vi "CreateTriggerOutputNode.vi"(7 "DOM Document":refnum<k20>, 8 "Error In":errorcluster, 11 "Trigger Output Configuration":T1={"Type"=enum."None", "Delay (ms)"=0, "Digital IO Line (1-14)"=1, "Digital IO Mode"=enum."Falling", "Digital IO Pulse Width (sec)"=0.0001} {"Digital IO Line (1-14)" min=1 max=14 step=1}) -> (0 "Error Out":errorcluster, 3 "Trigger Output Node":refnum<k20>)   [LabVIEW 2012]
uses:
  TriggerOutputConfiguration.ctl
  TriggerOutputType.ctl
  driver/Public/Controls/TriggerMode.ctl
  libs/LV-Utilities/LV-Utilities.lvlib
  driver/Keithley-2602.lvlib
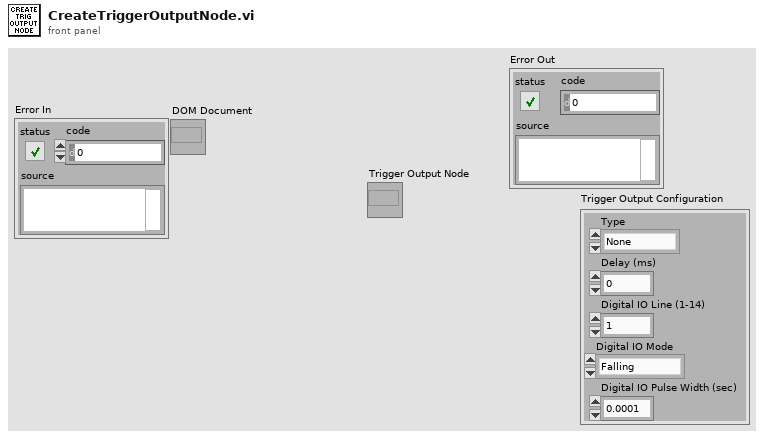
[diagram p1: front panel]
types:
  T1 = typedef "TriggerOutputConfiguration.ctl" = cluster{"Type":T2, "Delay (ms)":u32, "Digital IO Line (1-14)":u8, "Digital IO Mode":T3, "Digital IO Pulse Width (sec)":dbl}
  T2 = typedef "TriggerOutputType.ctl" = enum16{"None", "Digital IO", "Bus"}
  T3 = typedef "Keithley-2602.lvlib/TriggerMode.ctl" = enum16{"Falling", "Rising", "Either", "Synchronous"}
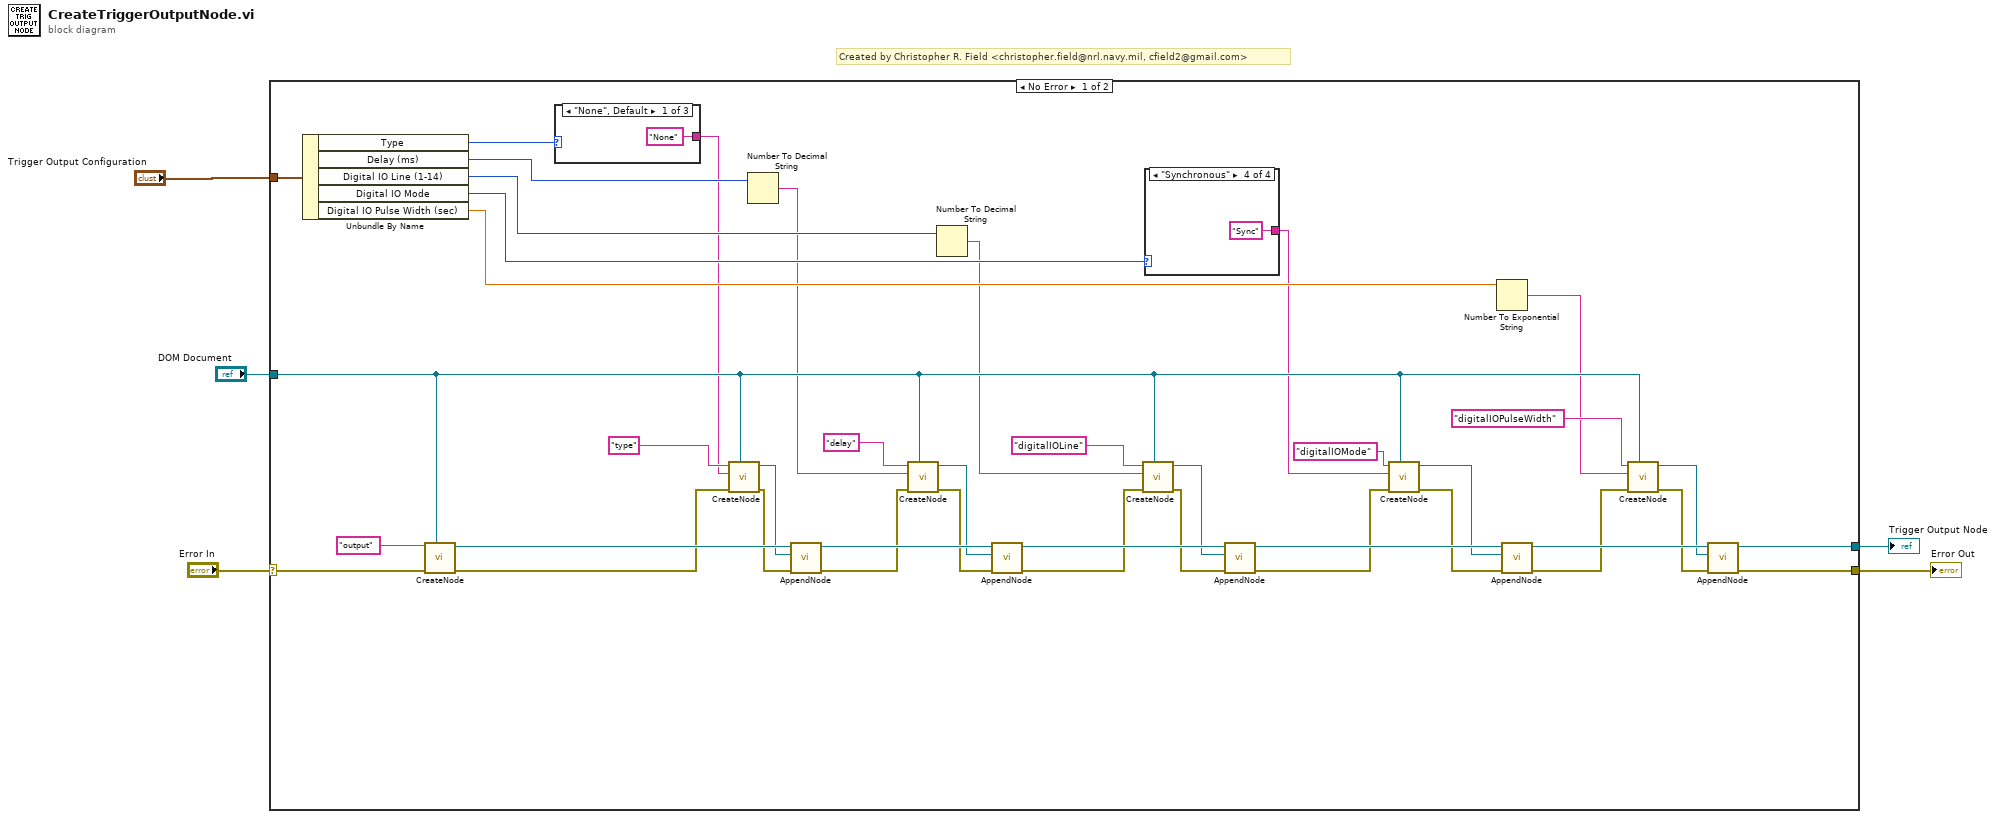
[diagram p0: block diagram]
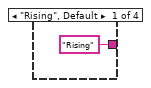
[diagram p2: hidden frame]
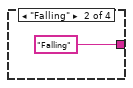
[diagram p3: hidden frame]
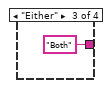
[diagram p4: hidden frame]
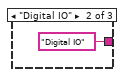
[diagram p5: hidden frame]
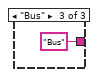
[diagram p6: hidden frame]
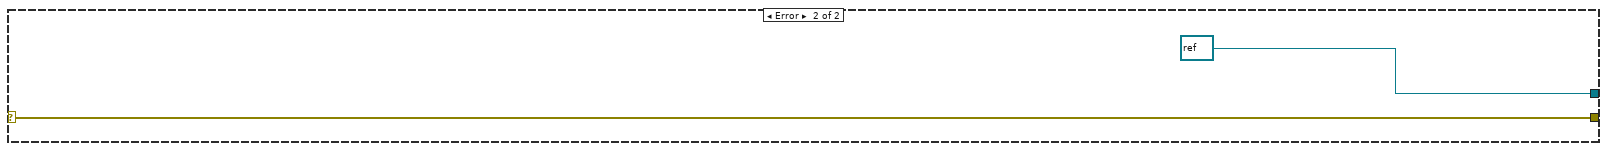
[diagram p7: hidden frame]
diagram:
  # "Created by Christopher R. Field <christopher.field@nrl.navy.mil, cfield2@gmail.com>"
  n1 = case shown="No Error" "Error In" {
    selector: "Error In" -> [w40 w55]
    tunnel: "DOM Document" -> [w26 _]
    tunnel: [w33 refnum<k20> refnum ("Wirings Node 2")] -> w3
    tunnel: [w32 w55] -> w2
    tunnel: "Trigger Output Configuration" -> [w45 _]
    frame No Error {
      n2 = Unbundle By Name(w45) -> ("Type"=w46:T2, "Delay (ms)"=w41:u32, "Digital IO Line (1-14)"=w44:u8, "Digital IO Mode"=w43:T3, "Digital IO Pulse Width (sec)"=w42:dbl)
      n3 = call "CreateNode.vi"("DOM Document"=w26, "Error In"=w40, "Tag Name"="output") -> ("Error out"=w25:errorcluster, "Node"=w38:refnum<k20>)  [unwired: 7 in]
      n4 = case shown="\"None\", Default" w46 {
        tunnel: ["None" "Digital IO" "Bus"] -> w10
        frame "None", Default {
        }
        frame "Digital IO" {
        }
        frame "Bus" {
        }
      }
      n5 = call "CreateNode.vi"("DOM Document"=w26, "Error In"=w25, "Text"=w10, "Tag Name"="type") -> ("Error out"=w24:errorcluster, "Node"=w11:refnum<k20>)  [unwired: 6 in]
      n6 = Number To Decimal String(number=w41) -> (decimal integer string=w9:string)  [unwired: 1 in]
      n7 = call "AppendNode.vi"("Error In"=w24, "Child Node"=w11, "Parent Node In"=w38) -> ("Error Out"=w23:errorcluster, "Parent Node Out"=w37:refnum<k20>)  [unwired: 7 in]
      n8 = call "CreateNode.vi"("DOM Document"=w26, "Error In"=w23, "Text"=w9, "Tag Name"="delay") -> ("Error out"=w22:errorcluster, "Node"=w12:refnum<k20>)  [unwired: 6 in]
      n9 = Number To Decimal String(number=w44) -> (decimal integer string=w8:string)  [unwired: 1 in]
      n10 = call "AppendNode.vi"("Error In"=w22, "Child Node"=w12, "Parent Node In"=w37) -> ("Error Out"=w21:errorcluster, "Parent Node Out"=w36:refnum<k20>)  [unwired: 7 in]
      n11 = call "CreateNode.vi"("DOM Document"=w26, "Error In"=w21, "Text"=w8, "Tag Name"="digitalIOLine" ("Text")) -> ("Error out"=w20:errorcluster, "Node"=w13:refnum<k20>)  [unwired: 6 in]
      n12 = case shown="\"Synchronous\"" w43 {
        tunnel: ["Rising" "Falling" "Both" "Sync"] -> w7
        frame "Rising", Default {
        }
        frame "Falling" {
        }
        frame "Either" {
        }
        frame "Synchronous" {
        }
      }
      n13 = call "AppendNode.vi"("Error In"=w20, "Child Node"=w13, "Parent Node In"=w36) -> ("Error Out"=w19:errorcluster, "Parent Node Out"=w35:refnum<k20>)  [unwired: 7 in]
      n14 = call "CreateNode.vi"("DOM Document"=w26, "Error In"=w19, "Text"=w7, "Tag Name"="digitalIOMode") -> ("Error out"=w18:errorcluster, "Node"=w14:refnum<k20>)  [unwired: 6 in]
      n15 = Number To Exponential String(number=w42) -> (E-format string=w6:string)  [unwired: 3 in]
      n16 = call "AppendNode.vi"("Error In"=w18, "Child Node"=w14, "Parent Node In"=w35) -> ("Error Out"=w17:errorcluster, "Parent Node Out"=w34:refnum<k20>)  [unwired: 7 in]
      n17 = call "CreateNode.vi"("DOM Document"=w26, "Error In"=w17, "Text"=w6, "Tag Name"="digitalIOPulseWidth") -> ("Error out"=w16:errorcluster, "Node"=w15:refnum<k20>)  [unwired: 6 in]
      n18 = call "AppendNode.vi"("Error In"=w16, "Child Node"=w15, "Parent Node In"=w34) -> ("Error Out"=w32:errorcluster, "Parent Node Out"=w33:refnum<k20>)  [unwired: 7 in]
    }
    frame Error {
    }
  }
  "Trigger Output Node" <- w3
  "Error Out" <- w2
